vi "neurona.vi"(0 "x1":dbl, 1 "x 2":dbl, 2 "w 1":dbl(slide) scale=-5.0..5.0, 3 "w 2":dbl(slide) scale=-5.0..5.0, 4 "B":dbl(slide) scale=-5.0..5.0) -> (5 "a":i16)   [LabVIEW 2016]
panel:
  out "XY Graph":cluster{dbl[], dbl[]}[](graph)
  out "x 2":dbl[](array[numeric])
  out "x1":dbl[](array[numeric])
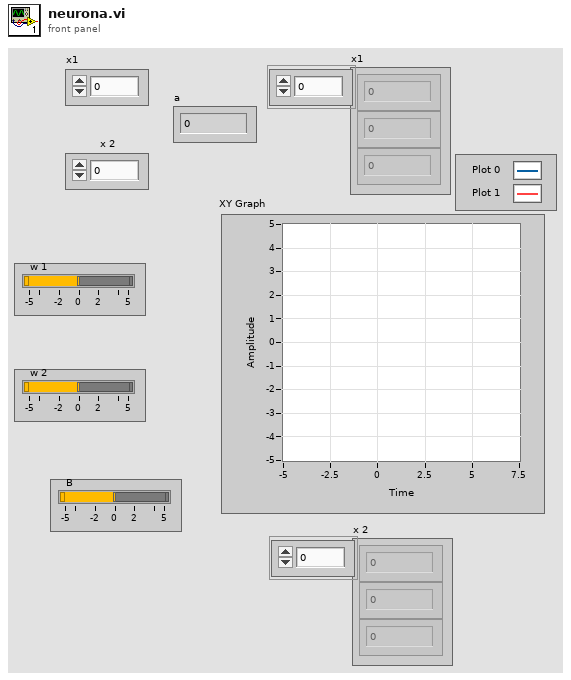
[diagram p1: front panel]
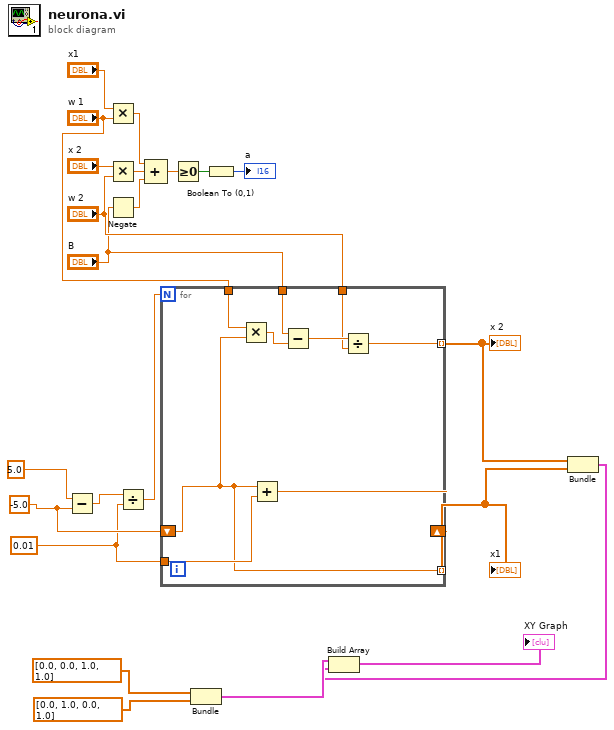
[diagram p0: block diagram]
diagram:
  w10 = 0.01
  w11 = -5.0
  n1 = Subtract(x=5.0, y=w11) -> (x-y=w13:dbl)
  n2 = Multiply(x="x1", y="w 1") -> (x*y=w21:dbl)
  n3 = Multiply(x="x 2", y="w 2") -> (x*y=w20:dbl)
  n4 = Negate(x="B") -> (-x=w9:dbl)
  n5 = Divide(x=w13, y=w10) -> (x/y=w12:dbl)
  n6 = Compound Arithmetic op=ADD(w21, w20, w9) -> (w19:dbl)
  n7 = for {
    N: w12 -> [_]
    shift-right: [w31] -> _
    shift-left: w11 -> [w29]
    tunnel: w10 -> [w32]
    tunnel: [w29] -> w6 mode=indexing
    tunnel: "w 1" -> [w30]
    tunnel: "w 2" -> [w26]
    tunnel: [w25] -> w5 mode=indexing
    tunnel: "B" -> [w24]
    n8 = Multiply(x=w30, y=w29) -> (x*y=w28:dbl)
    n9 = Add(x=w29, y=w32) -> (x+y=w31:dbl)
    n10 = Subtract(x=w24, y=w28) -> (x-y=w27:dbl)
    n11 = Divide(x=w27, y=w26) -> (x/y=w25:dbl)
  }
  "x1" <- w6
  "x 2" <- w5
  n12 = Greater Or Equal To 0?(x=w19) -> (x >= 0?=w18:bool)
  n13 = Bundle(dbl[] [0.0, 0.0, 1.0, 1.0], dbl[] [0.0, 1.0, 0.0, 1.0]) -> (w4:cluster{dbl[], dbl[]})  [unwired: 1 in]
  n14 = Boolean To (0,1)(Boolean=w18) -> (0, 1=→"a":i16)
  n15 = Bundle(w5, w6) -> (w3:cluster{dbl[], dbl[]})  [unwired: 1 in]
  n16 = Build Array(w4, w3) -> (→"XY Graph":cluster{dbl[], dbl[]}[])
